vi "FoundInstruments.vi"(8 "error in (no error)":errorcluster, 10 "Instruments Found":T1, 11 "Camera_Controller in":refnum<class "Camera_Controller.lvclass">) -> (0 "error out":errorcluster, 3 "Camera_Controller out":refnum<class "Camera_Controller.lvclass">)   [LabVIEW 2023, in "CameraLibrary.lvlib" / "Camera_Controller.lvlib" / "Camera_Controller.lvclass"]
uses:
  Camera_Controller.lvclass
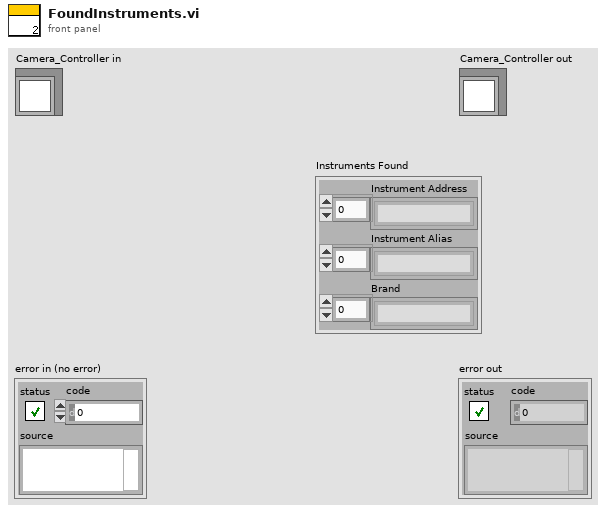
[diagram p1: front panel]
types:
  T1 = cluster{"Instrument Address":string[], "Instrument Alias":string[], "Brand":string[]}
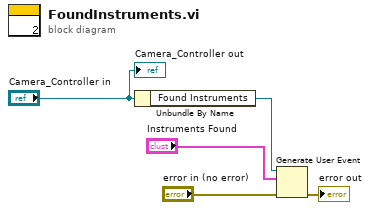
[diagram p0: block diagram]
diagram:
  n1 = Unbundle By Name("Camera_Controller in") -> ("Found Instruments"=w4:refnum<user-event>)
  n2 = Generate User Event(user event=w4, event data cluster="Instruments Found", error in="error in (no error)") -> (error out=→"error out":errorcluster)  [unwired: 1 in, 1 out]
  "Camera_Controller out" <- "Camera_Controller in"
